vi "Obtain Session.vi"(0 "SequenceFile":refnum<k7>, 2 "Engine":T1, 11 "error in (no error)":errorcluster, 12 "Skip Release? (F)":bool) -> (4 "Session Handle":T2, 15 "error out":errorcluster)   [LabVIEW 2020, in "TSS.lvlib" / "SequenceFile.lvclass"]
doc: "This function initializes the measurement\n\nPass the function a name to obtain an active measurement handle"
uses:
  SequenceFile.lvclass
  Typedefs/Session Handle.ctl
  C:/Program Files (x86)/National Instruments/LabVIEW 2020/user.lib/_Session Fwk/Session - Root.lvclass
  Engine/Typedefs/Session Handle.ctl
  Engine/Engine.lvclass
  SequenceFile.lvclass/SequenceFile.ctl
  <userlib>/_Session Fwk/Session - Root.lvclass
  TSS.lvlib
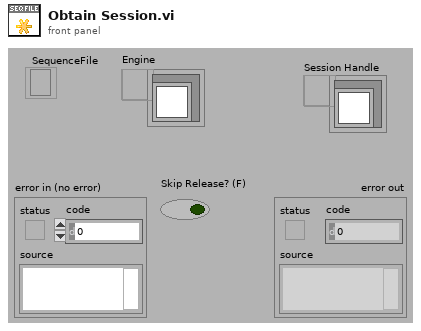
[diagram p1: front panel]
types:
  T1 = typedef "TSS.lvlib/Engine.lvclass/Session Handle.ctl" = refnum<data-value>
  T2 = typedef "TSS.lvlib/SequenceFile.lvclass/Session Handle.ctl" = refnum<data-value>
  T3 = typedef "TSS.lvlib/Sequence File Type.ctl" = enum16{"Normal", "Model", "Front End Callbacks", "Station Callbacks", "Template"}
  T4 = typedef "Session - Root.lvclass/Session Handle.ctl" = refnum<data-value>
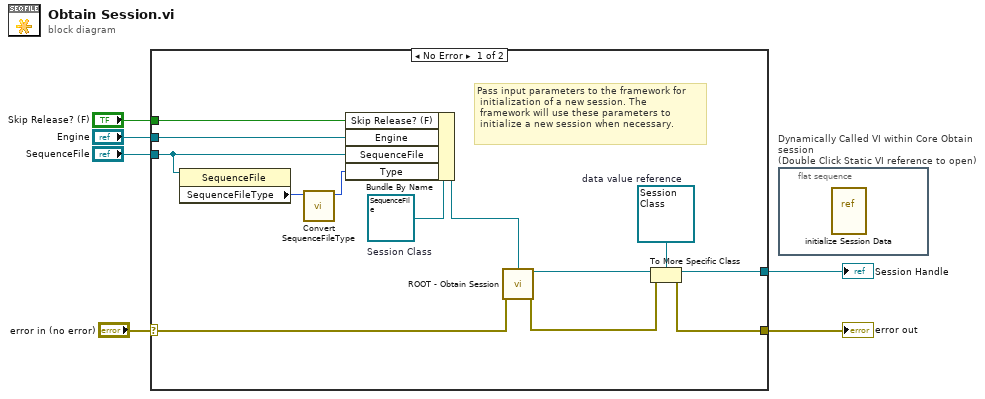
[diagram p0: block diagram]
diagram:
  n1 = case shown="No Error" "error in (no error)" {
    selector: "error in (no error)" -> [w19 w20]
    tunnel: [w16 w20] -> w5
    tunnel: [w18 _] -> w4
    tunnel: "SequenceFile" -> [w10 _]
    tunnel: "Engine" -> [w11 _]
    tunnel: "Skip Release? (F)" -> [w7 _]
    frame No Error {
      w12 = refnum<data-value> refnum  # data value reference
      w13 = refnum<class "SequenceFile.lvclass"> refnum  # Session Class
      # "Pass input parameters to the framework for\n initialization of a new session. The\n framework will use these parameters to\n initialize a new session when necessary."
      n2 = property class="SequenceFile"(reference=w10) -> ("SequenceFileType"=w9:i32)  [unwired: 1 in, 2 out]
      n3 = call "Convert SequenceFileType.vi"("API"=w9) -> ("API -> TSS"=w8:T3)  [unwired: 9 in, 1 out]
      n4 = Bundle By Name(cluster=w13, "Skip Release? (F)"=w7, "Engine"=w11, "SequenceFile"=w10, "Type"=w8) -> (w14:refnum<class "SequenceFile.lvclass">)
      n5 = call <userlib>:"ROOT - Obtain Session.vi"("OBJ - Session"=w14, "error in (no error)"=w19) -> ("Session Handle"=w15:T4, "error out"=w17:errorcluster)  [unwired: 11 in, 1 out]
      n6 = To More Specific Class(target class=w12, reference=w15, error in=w17) -> (specific class reference=w18:refnum<data-value>, error out=w16:errorcluster)
    }
    frame Error {
    }
  }
  "error out" <- w5
  "Session Handle" <- w4
  n7 = flat-sequence "Dynamically Called VI within Core Obtain session\n(Double Click Static VI reference to open)" {
    frame #0 {
      n8 = vi-ref "initialize Session Data.vi"() -> ()  [unwired: 1 out]
    }
  }
